vi "svi_write_zssp.vi"(4 "power value":dbl, 5 "position num":u32, 6 "shutter en entrée":bool, 7 "pdir_path":path, 9 "shutter 1":bool, 10 "z value":dbl, 11 "chanel num":u8) -> (0 "sortie d'erreur":errorcluster)   [LabVIEW 2013]
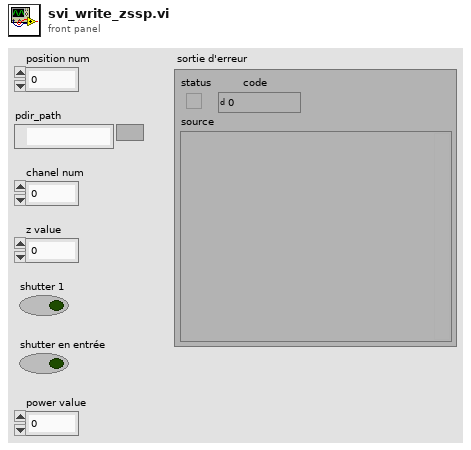
[diagram p1: front panel]
types:
  T1 = enum16{"open", "replace", "create", "open or create", "replace or create", "replace or create with confirmation"}
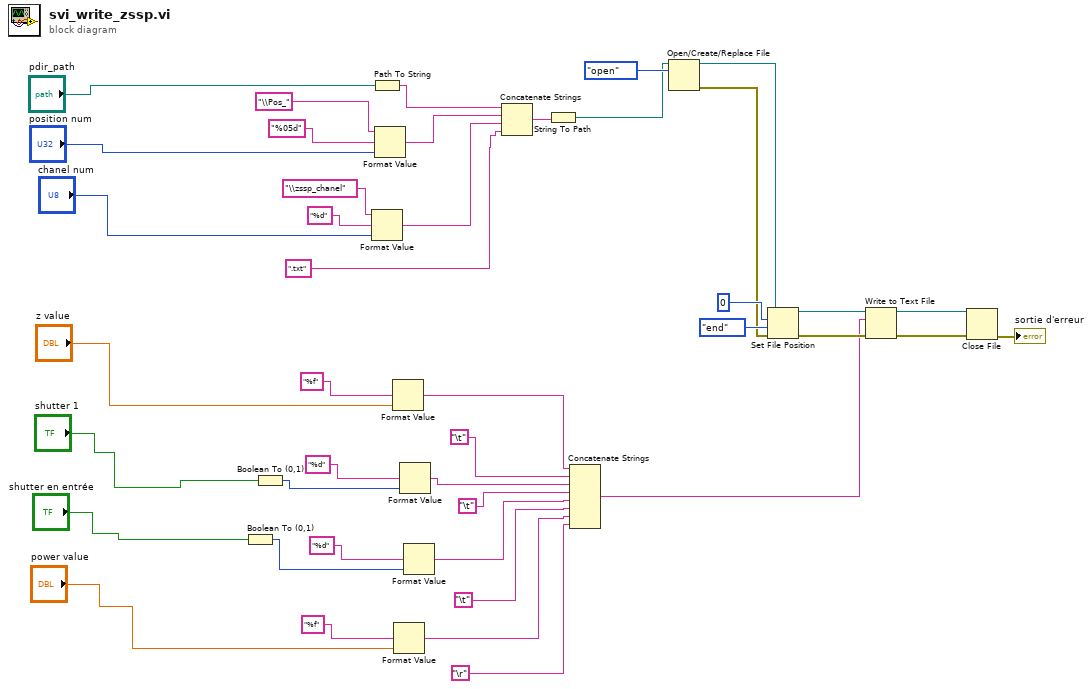
[diagram p0: block diagram]
diagram:
  n1 = Boolean To (0,1)(Boolean="shutter en entrée") -> (0, 1=w2:i16)
  n2 = Boolean To (0,1)(Boolean="shutter 1") -> (0, 1=w1:i16)
  n3 = Path To String(path="pdir_path") -> (string=w31:string)
  n4 = Format Value(string ("")="\\zssp_chanel", format string="%d" ("chaîne"), value (0)="chanel num") -> (output string=w29:string)
  n5 = Format Value(string ("")="\\Pos_", format string="%05d" ("chaîne"), value (0)="position num") -> (output string=w30:string)
  n6 = Format Value(format string="%f" ("chaîne"), value (0)="z value") -> (output string=w11:string)  [unwired: 1 in]
  n7 = Format Value(format string="%f" ("chaîne"), value (0)="power value") -> (output string=w5:string)  [unwired: 1 in]
  n8 = Format Value(format string="%d" ("chaîne"), value (0)=w1) -> (output string=w9:string)  [unwired: 1 in]
  n9 = Format Value(format string="%d" ("chaîne"), value (0)=w2) -> (output string=w7:string)  [unwired: 1 in]
  n10 = Concatenate Strings(w31, w30, w29, ".txt") -> (w26:string)
  n11 = String To Path(string=w26) -> (path=w25:path)
  n12 = Concatenate Strings(w11, "\t", w9, "\t", w7, "\t", w5, "\r") -> (w3:string)
  n13 = Open/Create/Replace File(file path (use dialog)=w25, operation (0:open)=T1."open") -> (refnum out=w22:refnum<file>, error out=w21:errorcluster)  [unwired: 4 in, 1 out]
  n14 = Set File Position(offset (in bytes) (0)=i64 0, refnum=w22, from (0:start)=enum16{"start", "end", "current"}."end", error in=w21) -> (refnum out=w19:refnum<file>, error out=w20:errorcluster)
  n15 = Write to Text File(file (use dialog)=w19, text=w3, error in=w20) -> (refnum out=w18:refnum<file>, error out=w17:errorcluster)  [unwired: 1 in, 1 out]
  n16 = Close File(refnum=w18, error in=w17) -> (error out=→"sortie d'erreur":errorcluster)  [unwired: 1 out]
